vi "message genarator.vi"(8 "error in":errorcluster, 10 "Message in":T2=enum."Welcome", 11 "Input data":string) -> (0 "error out":errorcluster, 1 "Left Menu":T1={"RFS String"="None", "RFS String 2"="Balance \nInquiry", "RFS String 3"="Return card\n& Terminate"}, 2 "Right Menu":T1={"RFS String"="Deposit", "RFS String 2"="Withdraw", "RFS String 3"="Fast Cash \n$50"}, 3 "Message out":string)   [LabVIEW 2015]
doc: "Generate proper message for any action"
uses:
  controls/message.ctl
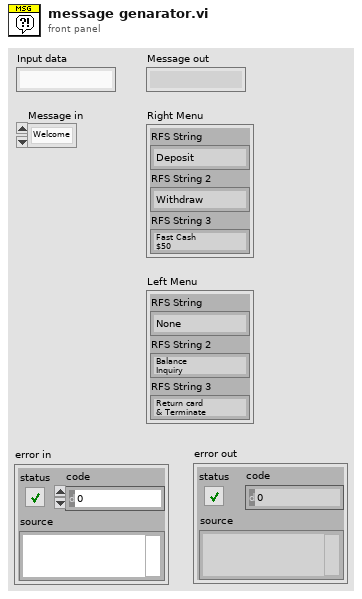
[diagram p1: front panel]
types:
  T1 = cluster{"RFS String":string, "RFS String 2":string, "RFS String 3":string}
  T2 = typedef "message.ctl" = enum16{"Deposit Complete", "Welcome", "Menu", "Verification Failed", "Session Terminate", "Deposit", "Withdrawal", "Withdrawal Complete", "Withdrawal Failed", "Balance Inq"}
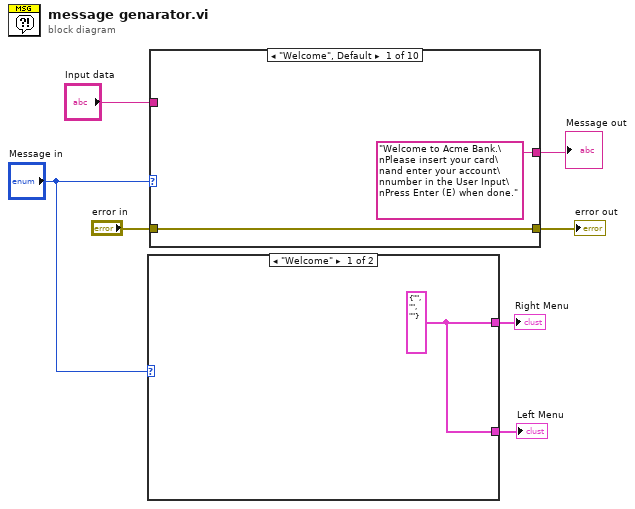
[diagram p0: block diagram]
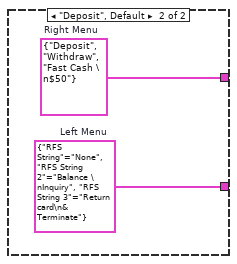
[diagram p2: hidden frame]
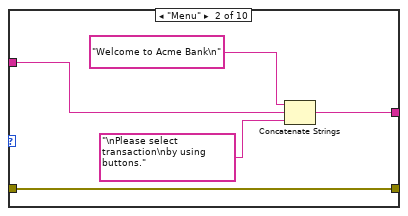
[diagram p3: hidden frame]
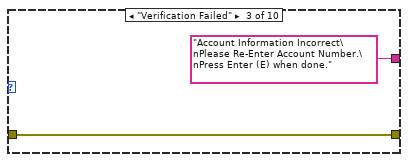
[diagram p4: hidden frame]
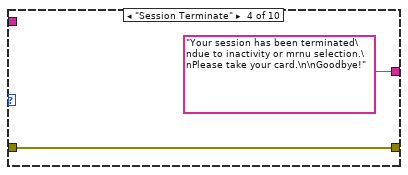
[diagram p5: hidden frame]
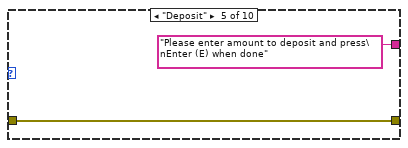
[diagram p6: hidden frame]
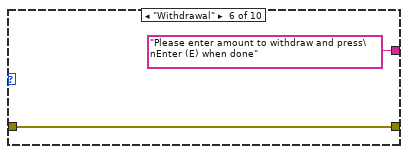
[diagram p7: hidden frame]
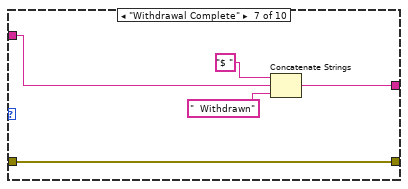
[diagram p8: hidden frame]
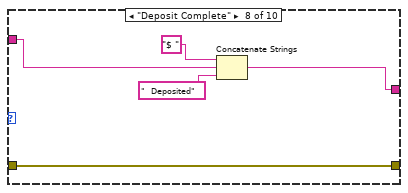
[diagram p9: hidden frame]
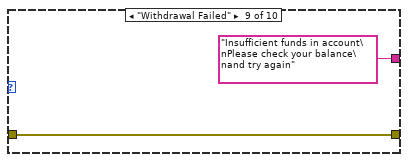
[diagram p10: hidden frame]
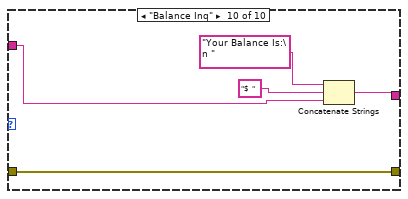
[diagram p11: hidden frame]
diagram:
  n1 = case shown="\"Welcome\"" "Message in" {
    tunnel: [w8 w10] -> w7
    tunnel: [w8 w9] -> w6
    frame "Welcome" {
      w8 = T1 {"RFS String"="", "RFS String 2"="", "RFS String 3"=""} ("Right Menu")
    }
    frame "Deposit", Default {
      w10 = T1 {"RFS String"="None", "RFS String 2"="Balance \nInquiry", "RFS String 3"="Return card\n& Terminate"}  # Left Menu
      w9 = T1 {"RFS String"="Deposit", "RFS String 2"="Withdraw", "RFS String 3"="Fast Cash \n$50"}  # Right Menu
    }
  }
  "Right Menu" <- w6
  "Left Menu" <- w7
  n2 = case shown="\"Welcome\", Default" "Message in" {
    tunnel: ["Welcome to Acme Bank.\nPlease insert your card\nand enter your account\nnumber in the User Input\nPress Enter (E) when done." w14 "Account Information Incorrect\nPlease Re-Enter Account Number.\nPress Enter (E) when done." "Your session has been terminated\ndue to inactivity or mrnu selection.\nPlease take your card.\n\nGoodbye!" "Please enter amount to deposit and press\nEnter (E) when done" "Please enter amount to withdraw and press\nEnter (E) when done" w27 w32 "Insufficient funds in account\nPlease check your balance\nand try again" w41] -> w4
    tunnel: "Input data" -> [_ w16 _ _ _ _ w28 w34 _ w39]
    tunnel: "error in" -> [w11 w13 w18 w20 w22 w24 w26 w31 w36 w38]
    tunnel: [w11 w13 w18 w20 w22 w24 w26 w31 w36 w38] -> w2
    frame "Welcome", Default {
    }
    frame "Menu" {
      n3 = Concatenate Strings("Welcome to Acme Bank\n", w16, "\nPlease select transaction\nby using buttons.") -> (w14:string)
    }
    frame "Verification Failed" {
    }
    frame "Session Terminate" {
    }
    frame "Deposit" {
    }
    frame "Withdrawal" {
    }
    frame "Withdrawal Complete" {
      n4 = Concatenate Strings("$ ", w28, "  Withdrawn" ("string")) -> (w27:string)
    }
    frame "Deposit Complete" {
      n5 = Concatenate Strings("$ ", w34, "  Deposited" ("string")) -> (w32:string)
    }
    frame "Withdrawal Failed" {
    }
    frame "Balance Inq" {
      n6 = Concatenate Strings("Your Balance Is:\n ", "$  " ("string"), w39) -> (w41:string)
    }
  }
  "Message out" <- w4
  "error out" <- w2
